vi "S4ACS.vi"() -> ()   [LabVIEW 2018]
uses:
  Channel Manager/Channel Manager.lvclass
  Channel/Channel.lvclass
panel:
  in  "Channels ID":u8=1
  in  "Software version":string="v1.12"
  in  "ACS Simulated/Real":bool
  in  "Number of channels":u8=1
  in  "Stop Button":bool
  out "Error Message":string
  in  "Channel Manager.lvclass":refnum<class "Channel Manager.lvclass">
  out "GUI Message":string
  out "ACS Message":string
  # "Welcome to the Acquisition Control System (ACS) of the SPARC4 instrument"
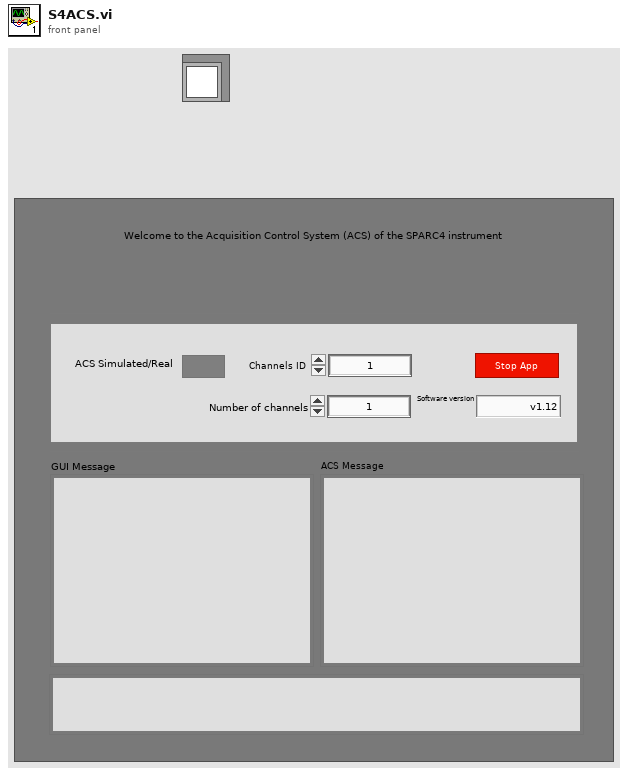
[diagram p1: front panel]
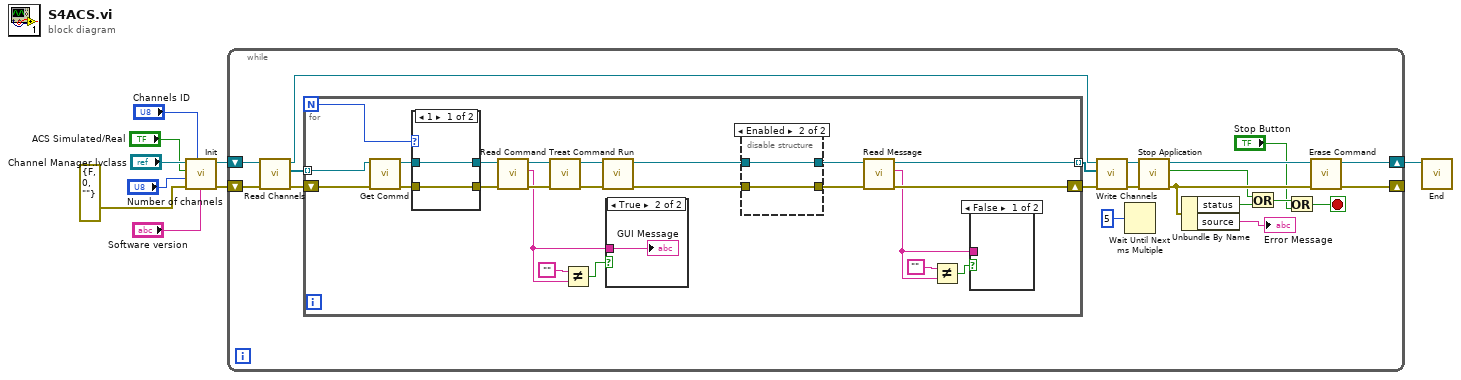
[diagram p0: block diagram]
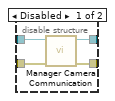
[diagram p2: hidden frame]
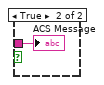
[diagram p3: hidden frame]
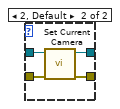
[diagram p4: hidden frame]
diagram:
  n1 = call "Init.vi"("Software version"="Software version", "Channels ID"="Channels ID", "error in (no error)"=errorcluster {"status"=FALSE, "code"=0, "source"=""}, "Channels quantity"="Number of channels", "ACS Simulated/Real"="ACS Simulated/Real", "Channel Manager in"="Channel Manager.lvclass") -> ("error out"=w8:errorcluster, "Channel Manager out"=w9:refnum<class "Channel Manager.lvclass">)  [unwired: 4 in]
  n2 = while {
    shift-right: [w11] -> _
    shift-left: w8 -> [w20]
    shift-right: [w18] -> w7
    shift-left: w9 -> [w21]
    stop <- w22 stop-if-true
    n3 = call "Read Channels.vi"("error in (no error)"=w20, "Channel Manager in"=w21) -> ("error out"=w29:errorcluster, "Array"=w15:refnum<class "Channel.lvclass">[], "Channel Manager out"=w27:refnum<class "Channel Manager.lvclass">)  [unwired: 7 in]
    n4 = for {
      N -> [w37]
      tunnel: w15 -> [w49] mode=indexing
      tunnel: [w34] -> w28 mode=indexing
      shift-right: [w33] -> w26
      shift-left: w29 -> [w50]
      n5 = call "Get Commd.vi"("error in (no error)"=w50, "Channel in"=w49) -> ("error out"=w43:errorcluster, "Channel out"=w44:refnum<class "Channel.lvclass">)  [unwired: 8 in]
      n6 = case shown="1" w37 {
        tunnel: [w60 w65] -> w52
        tunnel: [w61 w64] -> w51
        tunnel: w44 -> [w61 w63]
        tunnel: w43 -> [w60 w62]
        frame 1 {
        }
        frame 2, Default {
          n7 = call "Set Current Camera.vi"("error in (no error)"=w62, "Channel in"=w63) -> ("error out"=w65:errorcluster, "Channel out"=w64:refnum<class "Channel.lvclass">)  [unwired: 8 in]
        }
      }
      n8 = call "Read Command.vi"("error in (no error)"=w52, "Channel in"=w51) -> ("error out"=w46:errorcluster, "Message"=w41:string, "Channel out"=w47:refnum<class "Channel.lvclass">)  [unwired: 7 in]
      n9 = call "Treat Command.vi"("error in (no error)"=w46, "Channel in"=w47) -> ("error out"=w45:errorcluster, "Channel out"=w48:refnum<class "Channel.lvclass">)  [unwired: 8 in]
      n10 = Not Equal?(x="", y=w41) -> (x != y?=w42:bool)
      n11 = call "Run.vi"("error in (no error)"=w45, "Channel in"=w48) -> ("error out"=w39:errorcluster, "Channel out"=w38:refnum<class "Channel.lvclass">)  [unwired: 8 in]
      n12 = case shown="True" w42 {
        tunnel: w41 -> [_ w66]
        frame False {
        }
        frame True {
          "GUI Message" <- w66
        }
      }
      n13 = disable-structure shown="Enabled" {
        disable-tunnel: w39 -> [w56 w57]
        disable-tunnel: w38 -> [w55 w58]
        disable-tunnel: [w54 w57] -> w36
        disable-tunnel: [w53 w58] -> w35
        frame Disabled {
          n14 = call "Manager Camera Communication.vi"("error in (no error)"=w56, "Channel in"=w55) -> ("error out"=w54:errorcluster, "Channel out"=w53:refnum<class "Channel.lvclass">)  [unwired: 8 in]
        }
        frame Enabled {
        }
      }
      n15 = call "Read Message.vi"("error in (no error)"=w36, "Channel in"=w35) -> ("error out"=w33:errorcluster, "Rx Message"=w31:string, "Channel out"=w34:refnum<class "Channel.lvclass">)  [unwired: 7 in]
      n16 = Not Equal?(x="", y=w31) -> (x != y?=w32:bool)
      n17 = case shown="False" w32 {
        tunnel: w31 -> [_ w59]
        frame False {
        }
        frame True {
          "ACS Message" <- w59
        }
      }
    }
    n18 = call "Write Channels.vi"("error in (no error)"=w26, "Channels Array"=w28, "Channel Manager in"=w27) -> ("error out"=w25:errorcluster, "Channel Manager out"=w24:refnum<class "Channel Manager.lvclass">)  [unwired: 7 in]
    n19 = Wait Until Next ms Multiple(millisecond multiple=u32 5) -> ()  [unwired: 1 out]
    n20 = call "Stop Application.vi"("error in (no error)"=w25, "Channel Manager in"=w24) -> ("error out"=w17:errorcluster, "Stop Application"=w12:bool, "Channel Manager out"=w16:refnum<class "Channel Manager.lvclass">)  [unwired: 7 in]
    n21 = Unbundle By Name(w17) -> ("status"=w10:bool, "source"=→"Error Message":string)
    n22 = Or(x=w12, y=w10) -> (x .or. y?=w23:bool)
    n23 = Or(x=w23, y="Stop Button") -> (x .or. y?=w22:bool)
    n24 = call "Erase Command.vi"("error in (no error)"=w17, "Channel Manager in"=w16) -> ("error out"=w11:errorcluster, "Channel Manager out"=w18:refnum<class "Channel Manager.lvclass">)  [unwired: 8 in]
  }
  n25 = call "End.vi"("Channel Manager in"=w7) -> ()  [unwired: 9 in, 2 out]
